vi "Clave.vi"() -> ()   [LabVIEW 2015]
panel:
  in  "stop":bool
  out "String":string
  out "Clave":i32[](array[numeric])
  in  "OK":bool
  in  "0":bool
  in  "Clear":bool
  in  "3":bool
  in  "2":bool
  in  "1":bool
  in  "6":bool
  in  "5":bool
  in  "4":bool
  in  "9":bool
  in  "8":bool
  in  "7":bool
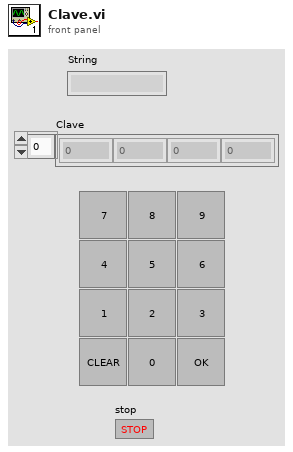
[diagram p1: front panel]
types:
  T1 = enum16{"Clave1", "Clave2", "Clave3", "Clave4", "Confirmación", "Default", ""}
  T2 = enum16{"Clave1", "Clave2", "Clave3", "Clave4", "Confirmación", "Default", ""}[]
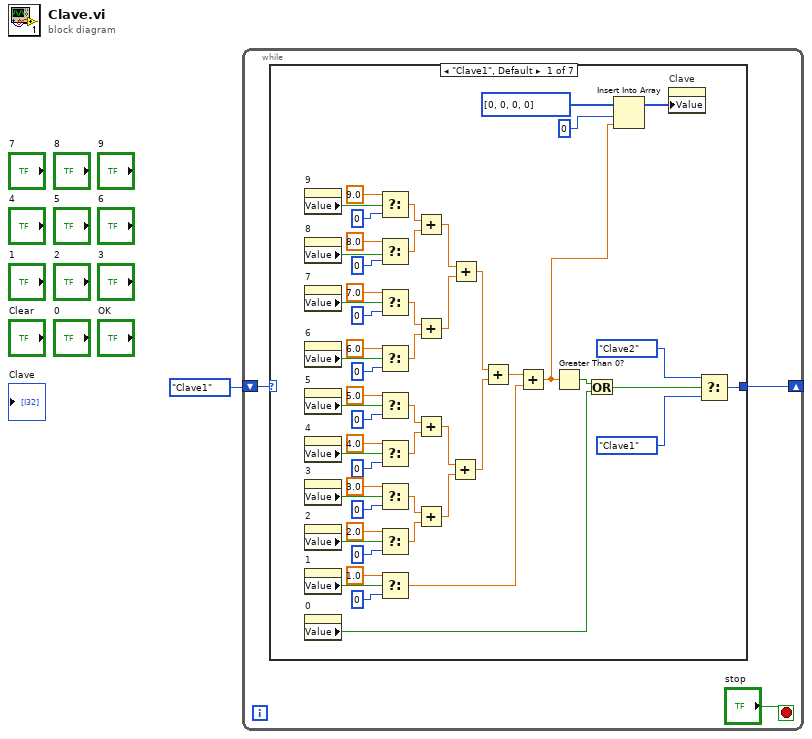
[diagram p0: block diagram]
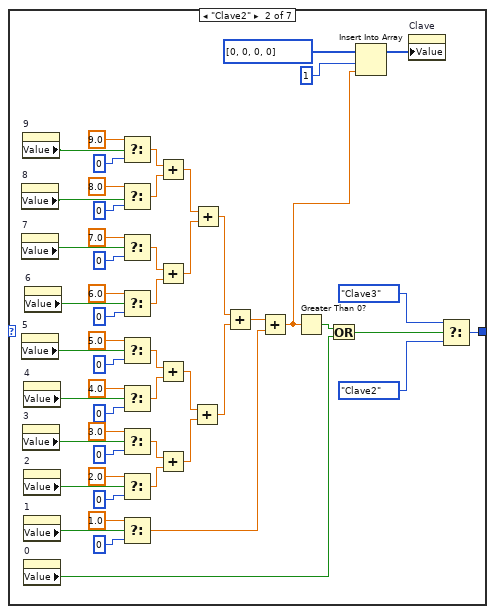
[diagram p2: hidden frame]
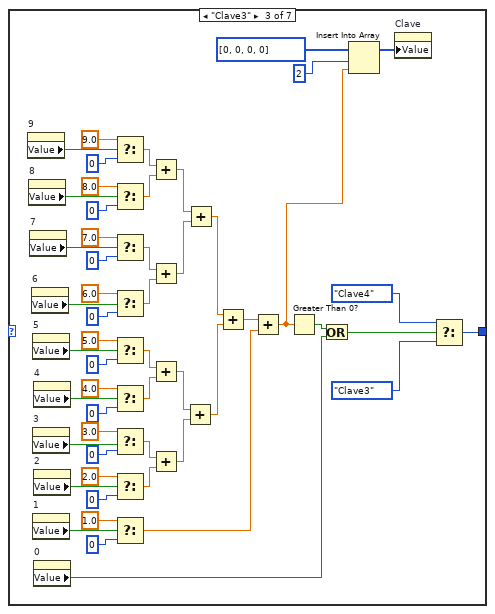
[diagram p3: hidden frame]
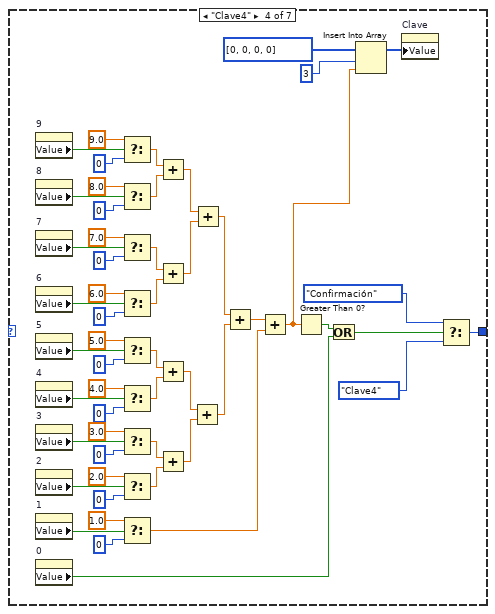
[diagram p4: hidden frame]
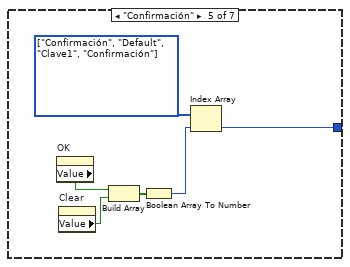
[diagram p5: hidden frame]
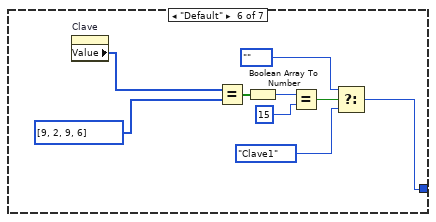
[diagram p6: hidden frame]
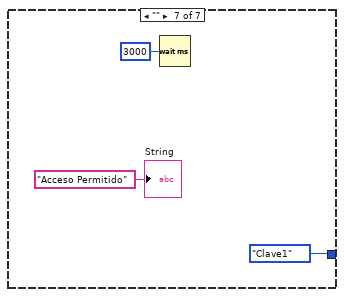
[diagram p7: hidden frame]
diagram:
  n1 = while {
    shift-right: [w4] -> _
    shift-left: T1."Clave1" -> [w3]
    stop <- "stop" stop-if-true
    n2 = case shown="\"Clave1\", Default" w3 {
      tunnel: [w6 w69 w122 w175 w217 w223 T1."Clave1"] -> w4
      frame "Clave1", Default {
        n3 = property on="9" class="Bool (strict)"() -> ("Value"=w55:bool)  [unwired: 2 in, 2 out]
        n4 = property on="8" class="Bool (strict)"() -> ("Value"=w54:bool)  [unwired: 2 in, 2 out]
        n5 = property on="7" class="Bool (strict)"() -> ("Value"=w53:bool)  [unwired: 2 in, 2 out]
        n6 = property on="6" class="Bool (strict)"() -> ("Value"=w52:bool)  [unwired: 2 in, 2 out]
        n7 = property on="5" class="Bool (strict)"() -> ("Value"=w51:bool)  [unwired: 2 in, 2 out]
        n8 = property on="4" class="Bool (strict)"() -> ("Value"=w50:bool)  [unwired: 2 in, 2 out]
        n9 = property on="3" class="Bool (strict)"() -> ("Value"=w49:bool)  [unwired: 2 in, 2 out]
        n10 = property on="2" class="Bool (strict)"() -> ("Value"=w48:bool)  [unwired: 2 in, 2 out]
        n11 = property on="1" class="Bool (strict)"() -> ("Value"=w47:bool)  [unwired: 2 in, 2 out]
        n12 = property on="0" class="Bool (strict)"() -> ("Value"=w11:bool)  [unwired: 2 in, 2 out]
        n13 = Select(t=9.0, s=w55, f=0 ("new element/subarray")) -> (s? t:f=w28:dbl)
        n14 = Select(t=8.0, s=w54, f=0 ("new element/subarray")) -> (s? t:f=w27:dbl)
        n15 = Select(t=7.0, s=w53, f=0 ("new element/subarray")) -> (s? t:f=w25:dbl)
        n16 = Select(t=6.0, s=w52, f=0 ("new element/subarray")) -> (s? t:f=w26:dbl)
        n17 = Select(t=5.0, s=w51, f=0 ("new element/subarray")) -> (s? t:f=w24:dbl)
        n18 = Select(t=4.0, s=w50, f=0 ("new element/subarray")) -> (s? t:f=w23:dbl)
        n19 = Select(t=3.0, s=w49, f=0 ("new element/subarray")) -> (s? t:f=w22:dbl)
        n20 = Select(t=2.0, s=w48, f=0 ("new element/subarray")) -> (s? t:f=w21:dbl)
        n21 = Select(t=1.0, s=w47, f=0 ("new element/subarray")) -> (s? t:f=w13:dbl)
        n22 = Add(x=w28, y=w27) -> (x+y=w20:dbl)
        n23 = Add(x=w25, y=w26) -> (x+y=w19:dbl)
        n24 = Add(x=w24, y=w23) -> (x+y=w18:dbl)
        n25 = Add(x=w22, y=w21) -> (x+y=w17:dbl)
        n26 = Add(x=w18, y=w17) -> (x+y=w15:dbl)
        n27 = Add(x=w20, y=w19) -> (x+y=w16:dbl)
        n28 = Add(x=w16, y=w15) -> (x+y=w14:dbl)
        n29 = Add(x=w14, y=w13) -> (x+y=w10:dbl)
        n30 = Greater Than 0?(x=w10) -> (x > 0?=w12:bool)
        n31 = Or(x=w12, y=w11) -> (x .or. y?=w9:bool)
        n32 = Insert Into Array(array=i32[] [0, 0, 0, 0], index=0, new element=w10) -> (w5:i32[])
        n33 = property on="Clave" class="Arr (strict)"("Value"=w5) -> ()  [unwired: 2 in, 2 out]
        n34 = Select(t=T1."Clave2", s=w9, f=T1."Clave1") -> (s? t:f=w6:T1)
      }
      frame "Clave2" {
        n35 = property on="8" class="Bool (strict)"() -> ("Value"=w67:bool)  [unwired: 2 in, 2 out]
        n36 = property on="7" class="Bool (strict)"() -> ("Value"=w66:bool)  [unwired: 2 in, 2 out]
        n37 = property on="5" class="Bool (strict)"() -> ("Value"=w64:bool)  [unwired: 2 in, 2 out]
        n38 = property on="9" class="Bool (strict)"() -> ("Value"=w68:bool)  [unwired: 2 in, 2 out]
        n39 = property on="3" class="Bool (strict)"() -> ("Value"=w62:bool)  [unwired: 2 in, 2 out]
        n40 = property on="4" class="Bool (strict)"() -> ("Value"=w63:bool)  [unwired: 2 in, 2 out]
        n41 = property on="2" class="Bool (strict)"() -> ("Value"=w61:bool)  [unwired: 2 in, 2 out]
        n42 = property on="1" class="Bool (strict)"() -> ("Value"=w60:bool)  [unwired: 2 in, 2 out]
        n43 = property on="0" class="Bool (strict)"() -> ("Value"=w59:bool)  [unwired: 2 in, 2 out]
        n44 = property on="6" class="Bool (strict)"() -> ("Value"=w65:bool)  [unwired: 2 in, 2 out]
        n45 = Select(t=9.0, s=w68, f=0 ("new element/subarray")) -> (s? t:f=w90:dbl)
        n46 = Select(t=8.0, s=w67, f=0 ("new element/subarray")) -> (s? t:f=w89:dbl)
        n47 = Select(t=7.0, s=w66, f=0 ("new element/subarray")) -> (s? t:f=w87:dbl)
        n48 = Select(t=6.0, s=w65, f=0 ("new element/subarray")) -> (s? t:f=w88:dbl)
        n49 = Select(t=5.0, s=w64, f=0 ("new element/subarray")) -> (s? t:f=w86:dbl)
        n50 = Select(t=4.0, s=w63, f=0 ("new element/subarray")) -> (s? t:f=w85:dbl)
        n51 = Select(t=3.0, s=w62, f=0 ("new element/subarray")) -> (s? t:f=w84:dbl)
        n52 = Select(t=2.0, s=w61, f=0 ("new element/subarray")) -> (s? t:f=w83:dbl)
        n53 = Select(t=1.0, s=w60, f=0 ("new element/subarray")) -> (s? t:f=w75:dbl)
        n54 = Add(x=w90, y=w89) -> (x+y=w82:dbl)
        n55 = Add(x=w87, y=w88) -> (x+y=w81:dbl)
        n56 = Add(x=w86, y=w85) -> (x+y=w80:dbl)
        n57 = Add(x=w84, y=w83) -> (x+y=w79:dbl)
        n58 = Add(x=w80, y=w79) -> (x+y=w77:dbl)
        n59 = Add(x=w82, y=w81) -> (x+y=w78:dbl)
        n60 = Add(x=w78, y=w77) -> (x+y=w76:dbl)
        n61 = Add(x=w76, y=w75) -> (x+y=w73:dbl)
        n62 = Greater Than 0?(x=w73) -> (x > 0?=w74:bool)
        n63 = Or(x=w74, y=w59) -> (x .or. y?=w72:bool)
        n64 = Insert Into Array(array=i32[] [0, 0, 0, 0], index=1, new element=w73) -> (w58:i32[])
        n65 = property on="Clave" class="Arr (strict)"("Value"=w58) -> ()  [unwired: 2 in, 2 out]
        n66 = Select(t=T1."Clave3", s=w72, f=T1."Clave2") -> (s? t:f=w69:T1)
      }
      frame "Clave3" {
        n67 = property on="9" class="Bool (strict)"() -> ("Value"=w121:bool)  [unwired: 2 in, 2 out]
        n68 = property on="8" class="Bool (strict)"() -> ("Value"=w120:bool)  [unwired: 2 in, 2 out]
        n69 = property on="7" class="Bool (strict)"() -> ("Value"=w119:bool)  [unwired: 2 in, 2 out]
        n70 = property on="6" class="Bool (strict)"() -> ("Value"=w118:bool)  [unwired: 2 in, 2 out]
        n71 = property on="5" class="Bool (strict)"() -> ("Value"=w117:bool)  [unwired: 2 in, 2 out]
        n72 = property on="3" class="Bool (strict)"() -> ("Value"=w115:bool)  [unwired: 2 in, 2 out]
        n73 = property on="1" class="Bool (strict)"() -> ("Value"=w113:bool)  [unwired: 2 in, 2 out]
        n74 = property on="4" class="Bool (strict)"() -> ("Value"=w116:bool)  [unwired: 2 in, 2 out]
        n75 = property on="2" class="Bool (strict)"() -> ("Value"=w114:bool)  [unwired: 2 in, 2 out]
        n76 = property on="0" class="Bool (strict)"() -> ("Value"=w112:bool)  [unwired: 2 in, 2 out]
        n77 = Select(t=9.0, s=w121, f=0 ("new element/subarray")) -> (s? t:f=w143:dbl)
        n78 = Select(t=8.0, s=w120, f=0 ("new element/subarray")) -> (s? t:f=w142:dbl)
        n79 = Select(t=7.0, s=w119, f=0 ("new element/subarray")) -> (s? t:f=w140:dbl)
        n80 = Select(t=6.0, s=w118, f=0 ("new element/subarray")) -> (s? t:f=w141:dbl)
        n81 = Select(t=5.0, s=w117, f=0 ("new element/subarray")) -> (s? t:f=w139:dbl)
        n82 = Select(t=4.0, s=w116, f=0 ("new element/subarray")) -> (s? t:f=w138:dbl)
        n83 = Select(t=3.0, s=w115, f=0 ("new element/subarray")) -> (s? t:f=w137:dbl)
        n84 = Select(t=2.0, s=w114, f=0 ("new element/subarray")) -> (s? t:f=w136:dbl)
        n85 = Select(t=1.0, s=w113, f=0 ("new element/subarray")) -> (s? t:f=w128:dbl)
        n86 = Add(x=w143, y=w142) -> (x+y=w135:dbl)
        n87 = Add(x=w140, y=w141) -> (x+y=w134:dbl)
        n88 = Add(x=w139, y=w138) -> (x+y=w133:dbl)
        n89 = Add(x=w137, y=w136) -> (x+y=w132:dbl)
        n90 = Add(x=w133, y=w132) -> (x+y=w130:dbl)
        n91 = Add(x=w135, y=w134) -> (x+y=w131:dbl)
        n92 = Add(x=w131, y=w130) -> (x+y=w129:dbl)
        n93 = Add(x=w129, y=w128) -> (x+y=w126:dbl)
        n94 = Greater Than 0?(x=w126) -> (x > 0?=w127:bool)
        n95 = Or(x=w127, y=w112) -> (x .or. y?=w125:bool)
        n96 = Insert Into Array(array=i32[] [0, 0, 0, 0], index=2, new element=w126) -> (w111:i32[])
        n97 = property on="Clave" class="Arr (strict)"("Value"=w111) -> ()  [unwired: 2 in, 2 out]
        n98 = Select(t=T1."Clave4", s=w125, f=T1."Clave3") -> (s? t:f=w122:T1)
      }
      frame "Clave4" {
        n99 = property on="9" class="Bool (strict)"() -> ("Value"=w174:bool)  [unwired: 2 in, 2 out]
        n100 = property on="8" class="Bool (strict)"() -> ("Value"=w173:bool)  [unwired: 2 in, 2 out]
        n101 = property on="7" class="Bool (strict)"() -> ("Value"=w172:bool)  [unwired: 2 in, 2 out]
        n102 = property on="6" class="Bool (strict)"() -> ("Value"=w171:bool)  [unwired: 2 in, 2 out]
        n103 = property on="5" class="Bool (strict)"() -> ("Value"=w170:bool)  [unwired: 2 in, 2 out]
        n104 = property on="4" class="Bool (strict)"() -> ("Value"=w169:bool)  [unwired: 2 in, 2 out]
        n105 = property on="3" class="Bool (strict)"() -> ("Value"=w168:bool)  [unwired: 2 in, 2 out]
        n106 = property on="2" class="Bool (strict)"() -> ("Value"=w167:bool)  [unwired: 2 in, 2 out]
        n107 = property on="1" class="Bool (strict)"() -> ("Value"=w166:bool)  [unwired: 2 in, 2 out]
        n108 = property on="0" class="Bool (strict)"() -> ("Value"=w165:bool)  [unwired: 2 in, 2 out]
        n109 = Select(t=9.0, s=w174, f=0 ("new element/subarray")) -> (s? t:f=w196:dbl)
        n110 = Select(t=8.0, s=w173, f=0 ("new element/subarray")) -> (s? t:f=w195:dbl)
        n111 = Select(t=7.0, s=w172, f=0 ("new element/subarray")) -> (s? t:f=w193:dbl)
        n112 = Select(t=6.0, s=w171, f=0 ("new element/subarray")) -> (s? t:f=w194:dbl)
        n113 = Select(t=5.0, s=w170, f=0 ("new element/subarray")) -> (s? t:f=w192:dbl)
        n114 = Select(t=4.0, s=w169, f=0 ("new element/subarray")) -> (s? t:f=w191:dbl)
        n115 = Select(t=3.0, s=w168, f=0 ("new element/subarray")) -> (s? t:f=w190:dbl)
        n116 = Select(t=2.0, s=w167, f=0 ("new element/subarray")) -> (s? t:f=w189:dbl)
        n117 = Select(t=1.0, s=w166, f=0 ("new element/subarray")) -> (s? t:f=w181:dbl)
        n118 = Add(x=w196, y=w195) -> (x+y=w188:dbl)
        n119 = Add(x=w193, y=w194) -> (x+y=w187:dbl)
        n120 = Add(x=w192, y=w191) -> (x+y=w186:dbl)
        n121 = Add(x=w190, y=w189) -> (x+y=w185:dbl)
        n122 = Add(x=w186, y=w185) -> (x+y=w183:dbl)
        n123 = Add(x=w188, y=w187) -> (x+y=w184:dbl)
        n124 = Add(x=w184, y=w183) -> (x+y=w182:dbl)
        n125 = Add(x=w182, y=w181) -> (x+y=w179:dbl)
        n126 = Greater Than 0?(x=w179) -> (x > 0?=w180:bool)
        n127 = Or(x=w180, y=w165) -> (x .or. y?=w178:bool)
        n128 = Insert Into Array(array=i32[] [0, 0, 0, 0], index=3, new element=w179) -> (w164:i32[])
        n129 = property on="Clave" class="Arr (strict)"("Value"=w164) -> ()  [unwired: 2 in, 2 out]
        n130 = Select(t=T1."Confirmación", s=w178, f=T1."Clave4") -> (s? t:f=w175:T1)
      }
      frame "Confirmación" {
        w218 = T2 [enum."Confirmación", enum."Default", enum."Clave1", enum."Confirmación"] items=["Clave1", "Clave2", "Clave3", "Clave4", "Confirmación", "Default", ""]
        n131 = property on="OK" class="Bool (strict)"() -> ("Value"=w222:bool)  [unwired: 2 in, 2 out]
        n132 = property on="Clear" class="Bool (strict)"() -> ("Value"=w221:bool)  [unwired: 2 in, 2 out]
        n133 = Build Array(w222, w221) -> (w220:bool[])
        n134 = Boolean Array To Number(Boolean array=w220) -> (number=w219:u32)
        n135 = Index Array(array=w218, index=w219) -> (element=w217:T1)
      }
      frame "Default" {
        n136 = property on="Clave" class="Arr (strict)"() -> ("Value"=w231:i32[])  [unwired: 2 in, 2 out]
        n137 = Equal?(x=w231, y=i32[] [9, 2, 9, 6]) -> (x = y?=w229:bool[])
        n138 = Boolean Array To Number(Boolean array=w229) -> (number=w228:u32)
        n139 = Equal?(x=w228, y=u32 15) -> (x = y?=w226:bool)
        n140 = Select(t=T1."", s=w226, f=T1."Clave1") -> (s? t:f=w223:T1)
      }
      frame "" {
        n141 = Wait (ms)(milliseconds to wait=u32 3000) -> ()  [unwired: 1 out]
        "String" <- "Acceso Permitido" ("String")
      }
    }
  }
